vi "水样测试.vi"(10 "数据标记表":string(combo)="N", 11 "水样测试时间":dbl=1.0) -> ()   [LabVIEW 2016, in "斯坦道多参数.lvlib"]
panel:
  out "运行状态":u16(ring) items=["空闲", "水样测试", "标样核查"]
  out "多参数运行日志":string
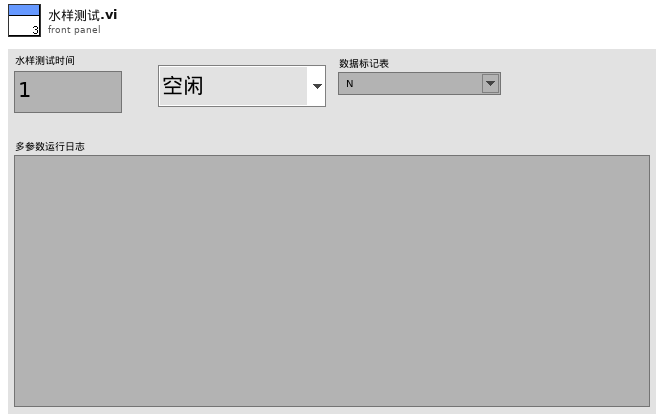
[diagram p1: front panel]
types:
  T1 = cluster{"因子编码":string, "单位":string, "标样参考值":sgl, "水样数据时间":timestamp, "水样实测值":sgl, "水样数据标识":string, "探头温度":sgl}
  T2 = cluster{"CH":u16, "监测值":dbl, "监测信号值":dbl, "温度偏移修正值":sgl}
  T3 = cluster{"电极状态标志":u16, "电极型号标志":u16, "酸碱度测量值":sgl, "温度测量值":sgl, "酸碱度信号值":sgl, "温度信号值":sgl, "酸碱度偏移修正值":sgl, "温度偏移修正值":sgl, "手动温度补偿值":sgl, "酸碱度电极零点":sgl, "酸碱度电极斜率":sgl, "第1点标准值记录":sgl, "第1点信号值记录":sgl, "第1点温度值记录":sgl, "第2点标准值记录":sgl, "第2点信号值记录":sgl, "第2点温度值记录":sgl, "命令滤波设定":u16, "温度模式":enum16{"ATC", "MTC"}, "生产批次":u16, "电极序号":u16, "串口地址":u16, "串口波特率":enum16{"9600", "19200", "115200"}, "串口校验位":enum16{"NONE", "ODD", "EVEN"}, "串口停止位":enum16{"1bit", "2bit"}, "第一点标准值":sgl, "第二点标准值":sgl}
  T4 = cluster{"电极状态标志":u16, "电极型号标志":u16, "电导率测量值":sgl, "温度测量值":sgl, "电导率信号值":sgl, "温度信号值":sgl, "温度补偿系数":sgl, "电导率偏移修正值":sgl, "温度偏移修正值":sgl, "手动温度补偿值":sgl, "电导率电极零点":sgl, "电导率电极斜率":sgl, "命令滤波设定":u16, "温度模式":enum16{"ATC", "MTC"}, "生产批次":u16, "电极序号":u16, "串口地址":u16, "串口波特率":enum16{"9600", "19200", "115200"}, "串口校验位":enum16{"NONE", "ODD", "EVEN"}, "串口停止位":enum16{"1bit", "2bit"}, "第一点标准值":sgl, "第二点标准值":sgl}
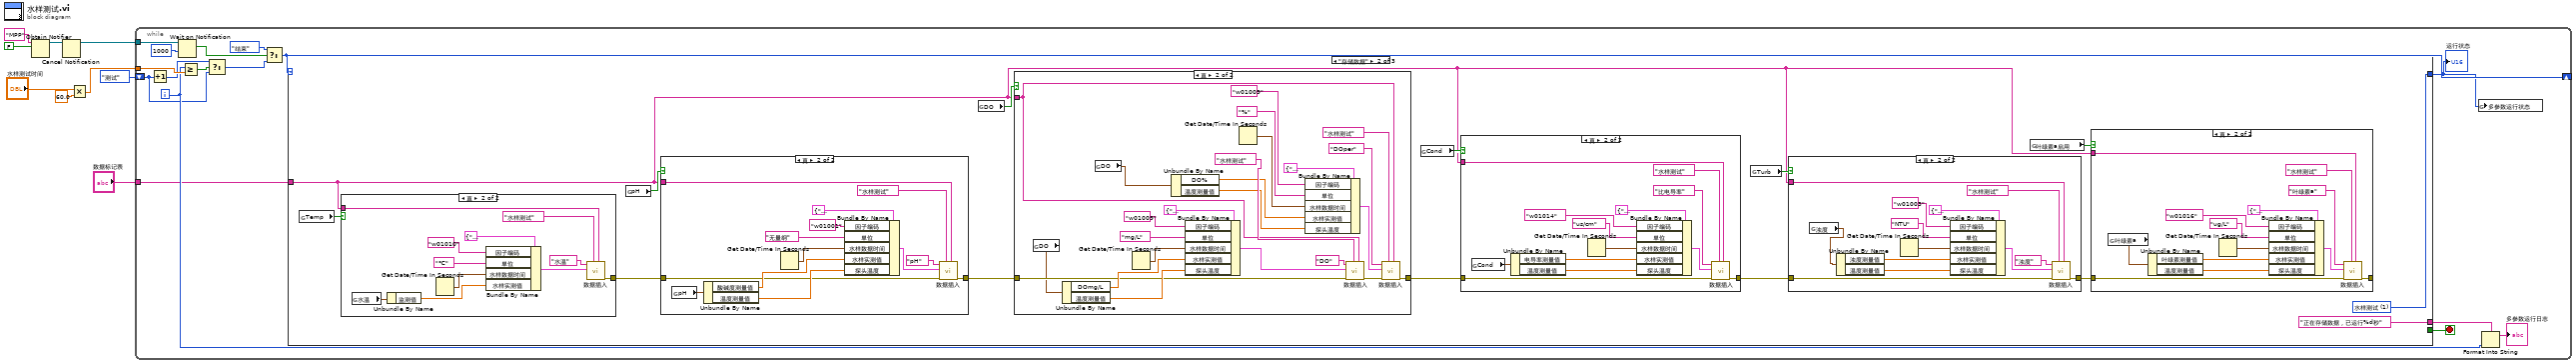
[diagram p0: block diagram]
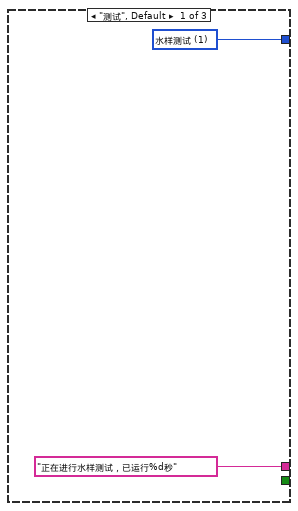
[diagram p2: hidden frame]
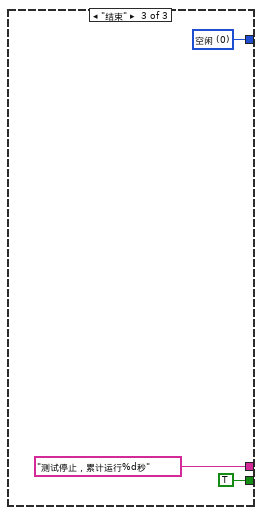
[diagram p9: hidden frame]
diagram:
  n1 = Obtain Notifier(name (unnamed)="MPP" ("名称（未命名）"), notification data type=FALSE) -> (notifier out=w3:refnum<notifier>)  [unwired: 2 in, 2 out]
  n2 = Cancel Notification(0:w3) -> (8:w2:refnum<notifier>)  [unwired: 1 in, 2 out]
  n3 = Multiply(x="水样测试时间", y=60.0) -> (x*y=w7:dbl)
  n4 = while {
    tunnel: w7 -> [w25]
    shift-right: [w12] -> _
    shift-left: enum16{"测试", "存储数据", "结束"}."测试" ("枚举") -> [w19]
    tunnel: w2 -> [w17]
    tunnel: "数据标记表" -> [w11]
    i -> [w23]
    stop <- w24 stop-if-true
    n5 = Increment(x=w19) -> (x+1=w18:enum16{"测试", "存储数据", "结束"})
    n6 = Wait on Notification(notifier=w17, timeout in ms (-1)=1000 ("超时毫秒(-1)")) -> (notification=w15:bool)  [unwired: 2 in, 3 out]
    n7 = Greater Or Equal?(x=w23, y=w25) -> (x >= y?=w20:bool)
    n8 = Select(t=w18, s=w20, f=w19) -> (s? t:f=w13:enum16{"测试", "存储数据", "结束"})
    n9 = Select(t=enum16{"测试", "存储数据", "结束"}."结束" ("枚举"), s=w15, f=w13) -> (s? t:f=w12:enum16{"测试", "存储数据", "结束"})
    n10 = case shown="\"存储数据\"" w12 {
      tunnel: [_ _ TRUE] -> w24
      tunnel: ["正在进行水样测试，已运行%d秒" ("格式字符串") "正在存储数据，已运行%d秒" ("格式字符串") "测试停止，累计运行%d秒" ("格式字符串")] -> w22
      tunnel: [w26 w29 w129] -> w10
      tunnel: w11 -> [_ w28 _]
      frame "测试", Default {
        w26 = u16 1 items=["空闲", "水样测试", "标样核查"] ("多参数运行状态")
      }
      frame "存储数据" {
        w29 = u16 1 items=["空闲", "水样测试", "标样核查"] ("多参数运行状态")
        n11 = global read "断电保存变量.vi" "Temp"() -> (w36:bool)
        n12 = case shown="真" w36 {
          tunnel: [_ w119] -> w31
          tunnel: w28 -> [_ w118]
          frame False {
          }
          frame True {
            n13 = global read "国弘过程全局变量.vi" "水温"() -> (w127:T2)
            n14 = Unbundle By Name(w127) -> ("监测值"=w126:dbl)
            n15 = Get Date/Time In Seconds() -> (seconds since 1Jan1904=w125:timestamp)
            n16 = Bundle By Name(cluster=T1 {"因子编码"="w01003", "单位"="无量纲", "标样参考值"=0.0, "水样数据时间"=timestamp(0 s since 1904-01-01), "水样实测值"=0.0, "水样数据标识"="N", "探头温度"=0.0} ("data in"), "因子编码"="w01010", "单位"="℃", "水样数据时间"=w125, "水样实测值"=w126) -> (w124:T1)
            n17 = call "数据插入.vi"("数据标记表"=w118, "测量模式"="水样测试", "data in"=w124, "table输入"="水温") -> ("error out"=w119:errorcluster)  [unwired: 7 in]
          }
        }
        n18 = global read "断电保存变量.vi" "pH"() -> (w37:bool)
        n19 = case shown="真" w37 {
          tunnel: w31 -> [_ w107]
          tunnel: [_ w106] -> w32
          tunnel: w28 -> [_ w105]
          frame False {
          }
          frame True {
            n20 = global read "国弘过程全局变量.vi" "pH"() -> (w113:T3)
            n21 = Unbundle By Name(w113) -> ("酸碱度测量值"=w114:sgl, "温度测量值"=w111:sgl)
            n22 = Get Date/Time In Seconds() -> (seconds since 1Jan1904=w115:timestamp)
            n23 = Bundle By Name(cluster=T1 {"因子编码"="w01003", "单位"="无量纲", "标样参考值"=0.0, "水样数据时间"=timestamp(0 s since 1904-01-01), "水样实测值"=0.0, "水样数据标识"="N", "探头温度"=0.0} ("data in"), "因子编码"="w01001", "单位"="无量纲", "水样数据时间"=w115, "水样实测值"=w114, "探头温度"=w111) -> (w116:T1)
            n24 = call "数据插入.vi"("数据标记表"=w105, "测量模式"="水样测试", "error in (no error)"=w107, "data in"=w116, "table输入"="pH") -> ("error out"=w106:errorcluster)  [unwired: 6 in]
          }
        }
        n25 = global read "断电保存变量.vi" "DO"() -> (w38:bool)
        n26 = case shown="真" w38 {
          tunnel: w32 -> [_ w95]
          tunnel: [_ w93] -> w33
          tunnel: w28 -> [_ w91]
          frame False {
          }
          frame True {
            n27 = global read "禹山过程全局变量.vi" "DO"() -> (w82:cluster{"温度测量值":sgl, "DO%":sgl, "DOmg/L":sgl})
            n28 = Unbundle By Name(w82) -> ("DOmg/L"=w102:sgl, "温度测量值"=w104:sgl)
            n29 = global read "禹山过程全局变量.vi" "DO"() -> (w81:cluster{"温度测量值":sgl, "DO%":sgl, "DOmg/L":sgl})
            n30 = Get Date/Time In Seconds() -> (seconds since 1Jan1904=w101:timestamp)
            n31 = Unbundle By Name(w81) -> ("DO%"=w86:sgl, "温度测量值"=w84:sgl)
            n32 = Bundle By Name(cluster=T1 {"因子编码"="w01003", "单位"="无量纲", "标样参考值"=0.0, "水样数据时间"=timestamp(0 s since 1904-01-01), "水样实测值"=0.0, "水样数据标识"="N", "探头温度"=0.0} ("data in"), "因子编码"="w01009", "单位"="mg/L", "水样数据时间"=w101, "水样实测值"=w102, "探头温度"=w104) -> (w100:T1)
            n33 = Get Date/Time In Seconds() -> (seconds since 1Jan1904=w87:timestamp)
            n34 = Bundle By Name(cluster=T1 {"因子编码"="w01003", "单位"="无量纲", "标样参考值"=0.0, "水样数据时间"=timestamp(0 s since 1904-01-01), "水样实测值"=0.0, "水样数据标识"="N", "探头温度"=0.0} ("data in"), "因子编码"="w01009", "单位"="%", "水样数据时间"=w87, "水样实测值"=w86, "探头温度"=w84) -> (w83:T1)
            n35 = call "数据插入.vi"("数据标记表"=w91, "测量模式"="水样测试", "error in (no error)"=w95, "data in"=w100, "table输入"="DO") -> ("error out"=w94:errorcluster)  [unwired: 6 in]
            n36 = call "数据插入.vi"("数据标记表"=w91, "测量模式"="水样测试", "error in (no error)"=w94, "data in"=w83, "table输入"="DOper") -> ("error out"=w93:errorcluster)  [unwired: 6 in]
          }
        }
        n37 = global read "断电保存变量.vi" "Cond"() -> (w39:bool)
        n38 = case shown="真" w39 {
          tunnel: w33 -> [_ w70]
          tunnel: [_ w69] -> w34
          tunnel: w28 -> [_ w68]
          frame False {
          }
          frame True {
            n39 = global read "国弘过程全局变量.vi" "Cond"() -> (w76:T4)
            n40 = Unbundle By Name(w76) -> ("电导率测量值"=w77:sgl, "温度测量值"=w74:sgl)
            n41 = Get Date/Time In Seconds() -> (seconds since 1Jan1904=w78:timestamp)
            n42 = Bundle By Name(cluster=T1 {"因子编码"="w01003", "单位"="无量纲", "标样参考值"=0.0, "水样数据时间"=timestamp(0 s since 1904-01-01), "水样实测值"=0.0, "水样数据标识"="N", "探头温度"=0.0} ("data in"), "因子编码"="w01014", "单位"="us/cm", "水样数据时间"=w78, "水样实测值"=w77, "探头温度"=w74) -> (w79:T1)
            n43 = call "数据插入.vi"("数据标记表"=w68, "测量模式"="水样测试", "error in (no error)"=w70, "data in"=w79, "table输入"="比电导率") -> ("error out"=w69:errorcluster)  [unwired: 6 in]
          }
        }
        n44 = global read "断电保存变量.vi" "Turb"() -> (w40:bool)
        n45 = case shown="真" w40 {
          tunnel: w34 -> [_ w58]
          tunnel: [_ w57] -> w35
          tunnel: w28 -> [_ w56]
          frame False {
          }
          frame True {
            n46 = global read "禹山过程全局变量.vi" "浊度"() -> (w55:cluster{"温度测量值":sgl, "浊度测量值":sgl})
            n47 = Unbundle By Name(w55) -> ("浊度测量值"=w65:sgl, "温度测量值"=w67:sgl)
            n48 = Get Date/Time In Seconds() -> (seconds since 1Jan1904=w64:timestamp)
            n49 = Bundle By Name(cluster=T1 {"因子编码"="w01003", "单位"="无量纲", "标样参考值"=0.0, "水样数据时间"=timestamp(0 s since 1904-01-01), "水样实测值"=0.0, "水样数据标识"="N", "探头温度"=0.0} ("data in"), "因子编码"="w01003", "单位"="NTU", "水样数据时间"=w64, "水样实测值"=w65, "探头温度"=w67) -> (w63:T1)
            n50 = call "数据插入.vi"("数据标记表"=w56, "测量模式"="水样测试", "error in (no error)"=w58, "data in"=w63, "table输入"="浊度") -> ("error out"=w57:errorcluster)  [unwired: 6 in]
          }
        }
        n51 = global read "断电保存变量.vi" "叶绿素a启用"() -> (w41:bool)
        n52 = case shown="真" w41 {
          tunnel: w35 -> [_ w45]
          tunnel: [_ w44] -> _
          tunnel: w28 -> [_ w43]
          frame False {
          }
          frame True {
            n53 = global read "禹山过程全局变量.vi" "叶绿素a"() -> (w42:cluster{"温度测量值":sgl, "叶绿素测量值":sgl, "错误标志":u16})
            n54 = Unbundle By Name(w42) -> ("叶绿素测量值"=w52:sgl, "温度测量值"=w50:sgl)
            n55 = Get Date/Time In Seconds() -> (seconds since 1Jan1904=w53:timestamp)
            n56 = Bundle By Name(cluster=T1 {"因子编码"="w01003", "单位"="无量纲", "标样参考值"=0.0, "水样数据时间"=timestamp(0 s since 1904-01-01), "水样实测值"=0.0, "水样数据标识"="N", "探头温度"=0.0} ("data in"), "因子编码"="w01016", "单位"="ug/L", "水样数据时间"=w53, "水样实测值"=w52, "探头温度"=w50) -> (w48:T1)
            n57 = call "数据插入.vi"("数据标记表"=w43, "测量模式"="水样测试", "error in (no error)"=w45, "data in"=w48, "table输入"="叶绿素a") -> ("error out"=w44:errorcluster)  [unwired: 6 in]
          }
        }
      }
      frame "结束" {
        w129 = u16 0 items=["空闲", "水样测试", "标样核查"] ("多参数运行状态")
      }
    }
    "运行状态" <- w10
    n58 = global write "多参数全局变量.vi" "多参数运行状态"(w10) -> ()
    n59 = Format Into String(format string=w22, w23) -> (resulting string=→"多参数运行日志":string)  [unwired: 2 in, 1 out]
  }
